vi "HMI Respirador.vi"() -> ()   [LabVIEW 2019]
uses:
  <vilib>/Instr/_visa.llb/VISA Configure Serial Port (Instr).vi
panel:
  in  "byte count":u32
  out "Waveform Chart":dynamicdata(graph)
  out "V. Espir.":bool
  out "V.Aspir":bool
  out "Boolean 3":bool
  out "Trama de Datos":string
  out "Meter":dbl(knob) scale=0.0..10.0
  out "VENTILADOR":bool
  out "TUBERIA EXHALACION":u8(slide)
  out "TUBERIA INHALACION":u8(slide) scale=0.0..115.0
  in  "stop":bool
  out "Velocidad Motor  R.P.M":i32
  out "Presion Entregada":i32
  in  "write buffer":string
  in  "Tiempo PEEP":u16
  out "read buffer":string
  out "Boolean":bool
  in  "Guardar Config":bool
  in  "Iniciar":bool
  in  "Puerto Comunicación":refnum<visa-resource-name>
  in  "Presión Maxima":u8
  in  "PEEP (pres. esp.)":u8
  in  "Tiempo Anspiracion":u16
  in  "Turbina %":u8
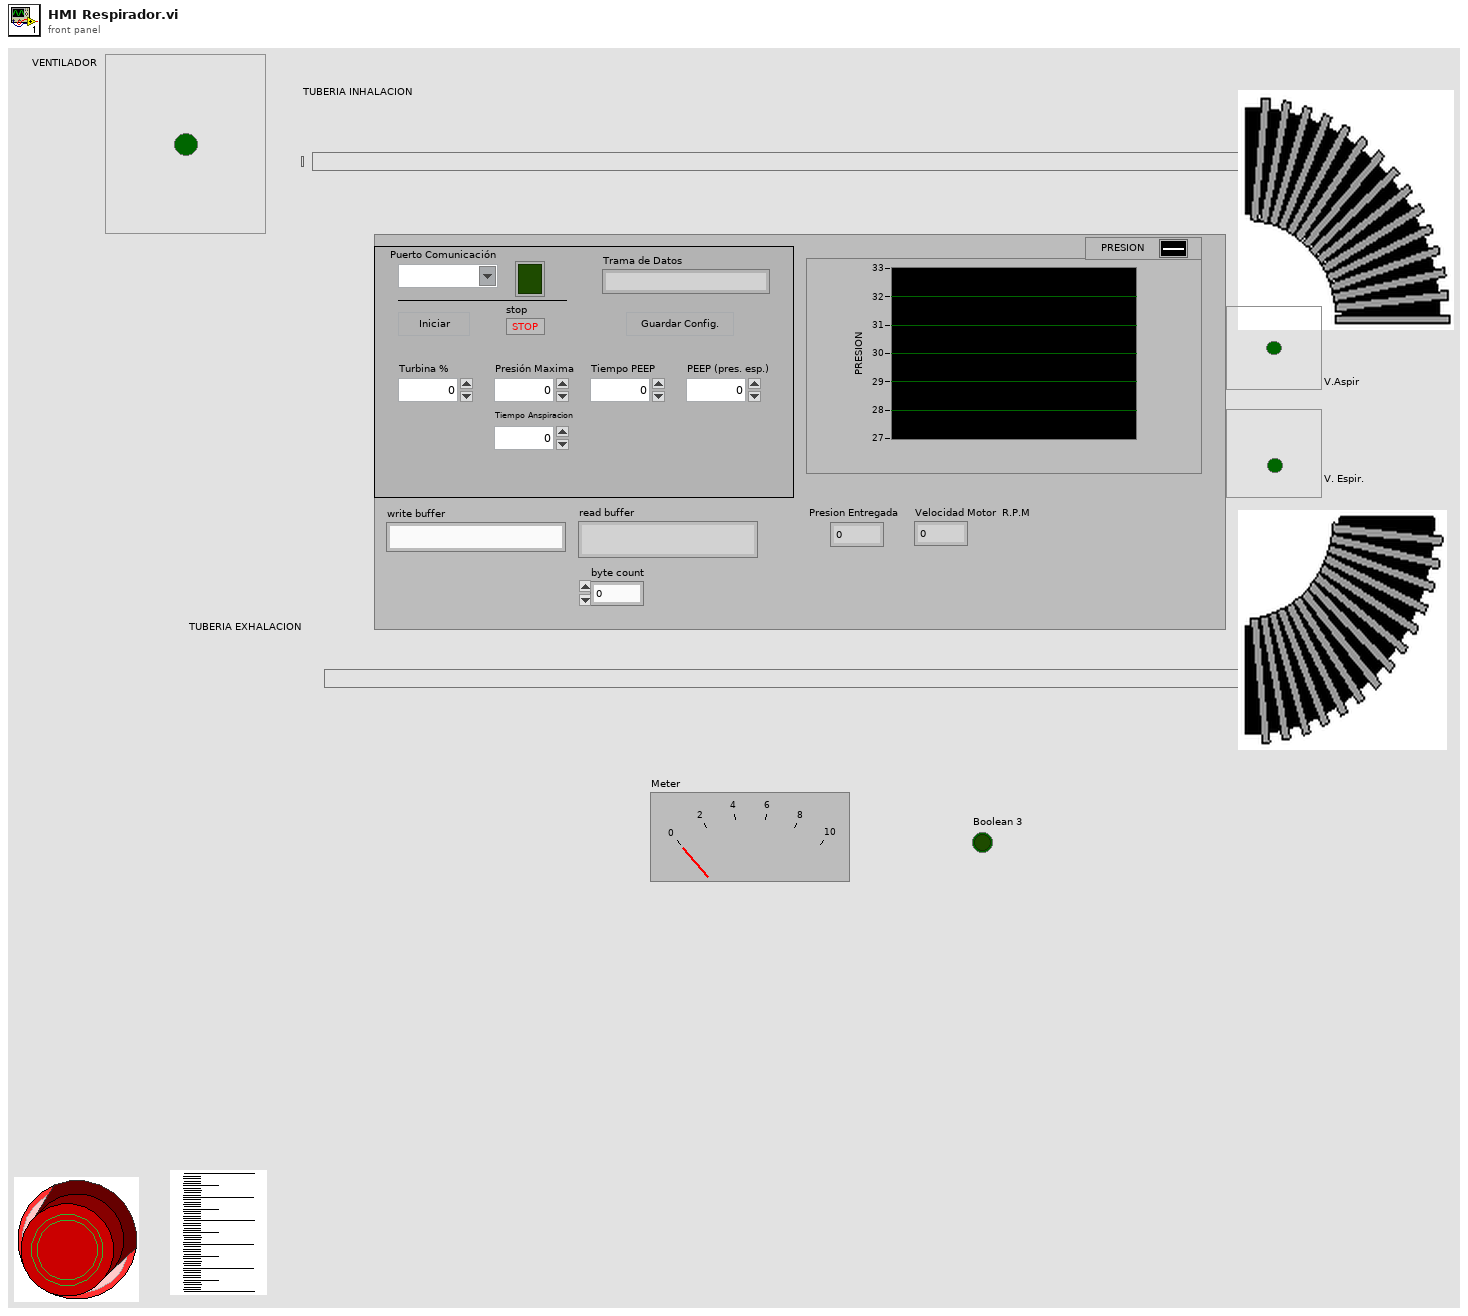
[diagram p1: front panel]
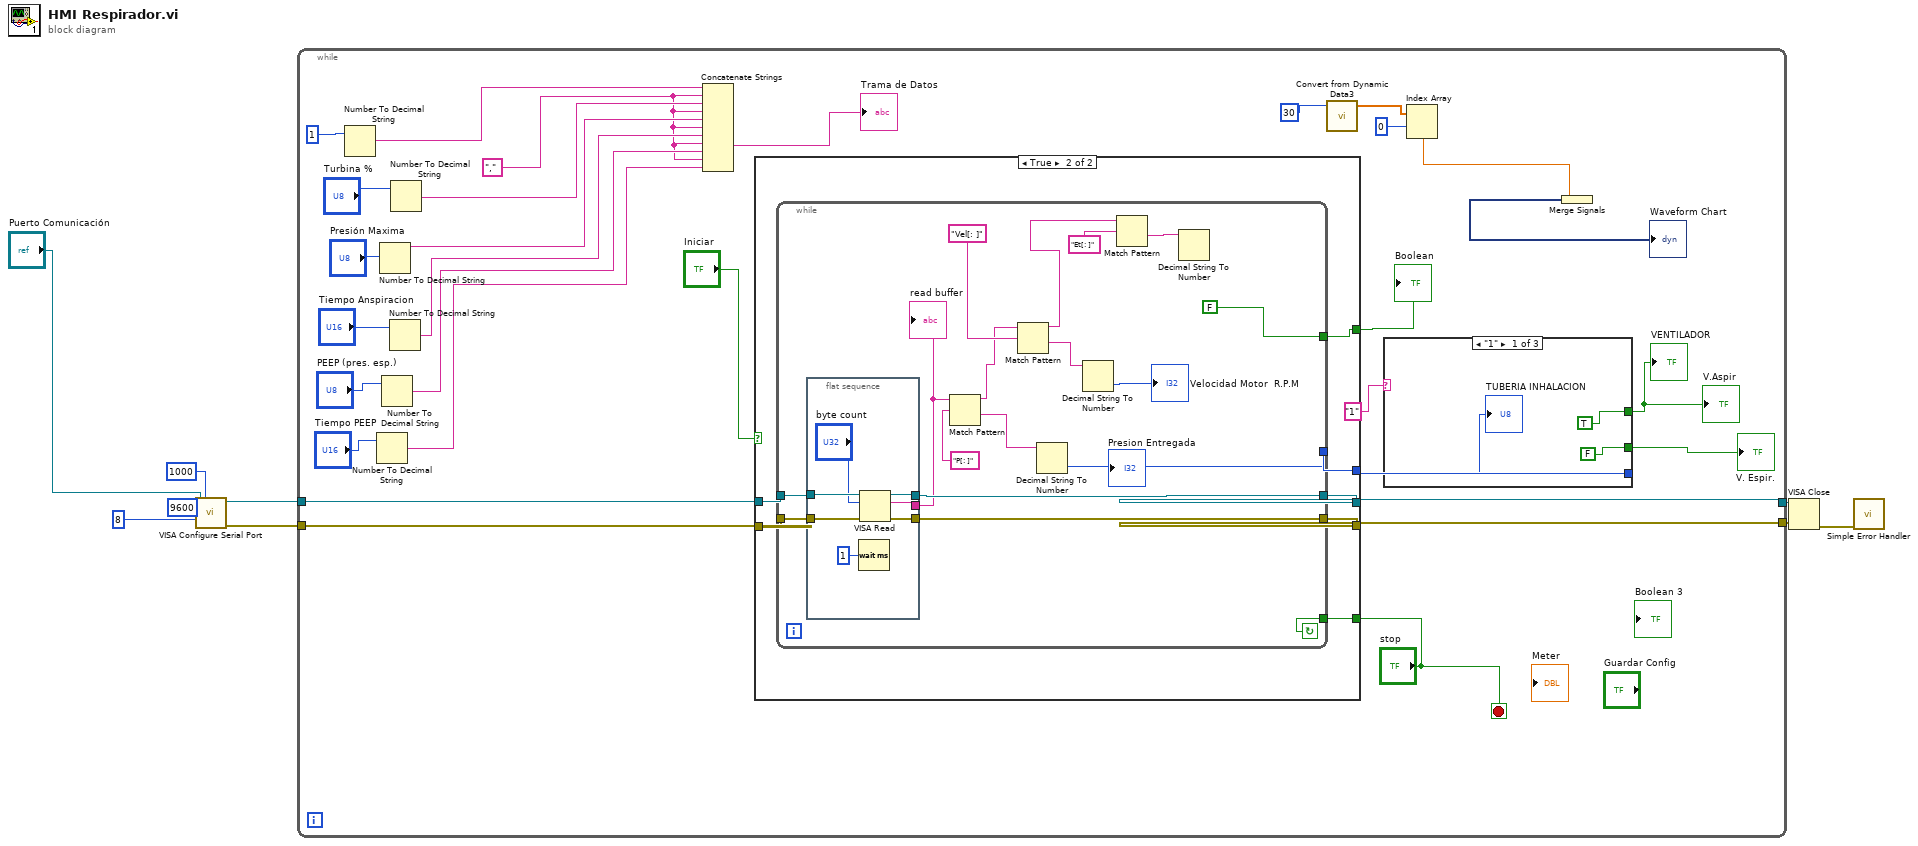
[diagram p0: block diagram]
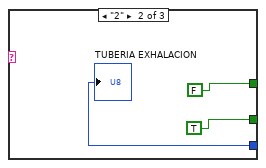
[diagram p2: hidden frame]
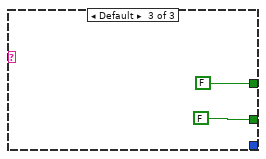
[diagram p3: hidden frame]
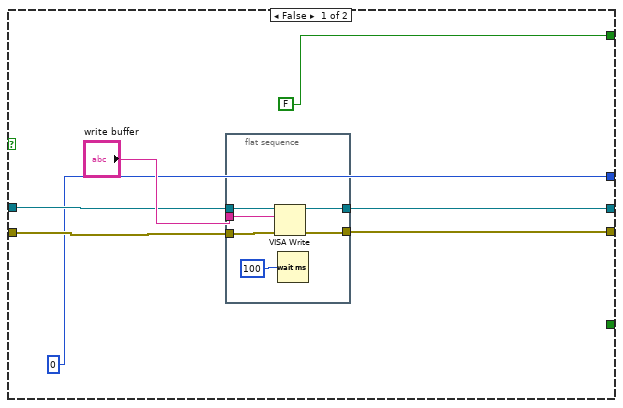
[diagram p4: hidden frame]
diagram:
  n1 = call-poly "VISA Configure Serial Port"("VISA resource name"="Puerto Comunicación", "timeout (10sec)"=u32 1000, "baud rate (9600)"=u32 9600, "data bits (8)"=u16 8) -> ("VISA resource name out"=w8:refnum<visa-resource-name>, "error out"=w7:errorcluster)  [unwired: 5 in, 5 out]
  n2 = while {
    tunnel: w8 -> [w37]
    tunnel: w7 -> [w38]
    tunnel: [w36] -> w4
    tunnel: [w35] -> w3
    stop <- "stop" stop-if-true
    w26 = ","
    n3 = Number To Decimal String(number=1) -> (decimal integer string=w31:string)  [unwired: 1 in]
    n4 = Number To Decimal String(number="Tiempo PEEP") -> (decimal integer string=w25:string)  [unwired: 1 in]
    n5 = Number To Decimal String(number="Presión Maxima") -> (decimal integer string=w29:string)  [unwired: 1 in]
    n6 = Number To Decimal String(number="PEEP (pres. esp.)") -> (decimal integer string=w27:string)  [unwired: 1 in]
    n7 = Number To Decimal String(number="Tiempo Anspiracion") -> (decimal integer string=w28:string)  [unwired: 1 in]
    n8 = Number To Decimal String(number="Turbina %") -> (decimal integer string=w30:string)  [unwired: 1 in]
    n9 = Concatenate Strings(w31, w26, w30, w26, w29, w26, w28, w26, w27, w26, w25) -> (→"Trama de Datos":string)
    n10 = case shown="True" "Iniciar" {
      tunnel: w37 -> [w51 w67]
      tunnel: w38 -> [w50 w66]
      tunnel: [w53 w65] -> w36
      tunnel: [w52 w64] -> w35
      tunnel: [FALSE w63] -> w23
      tunnel: "stop" -> [_ w62]
      tunnel: [0 w61] -> w18
      frame False {
        n11 = flat-sequence {
          tunnel: w51 -> [w60]
          tunnel: w50 -> [w59]
          tunnel: "write buffer" -> [w58]
          tunnel: [w57] -> w53
          tunnel: [w56] -> w52
          frame #0 {
            n12 = VISA Write(VISA resource name=w60, write buffer=w58, error in (no error)=w59) -> (VISA resource name out=w57:refnum<visa-resource-name>, error out=w56:errorcluster)  [unwired: 1 out]
            n13 = Wait (ms)(milliseconds to wait=u32 100) -> ()  [unwired: 1 out]
          }
        }
      }
      frame True {
        n14 = while {
          tunnel: w67 -> [w84]
          tunnel: [w82] -> w65
          tunnel: w66 -> [w83]
          tunnel: [w81] -> w64
          tunnel: [FALSE] -> w63
          tunnel: w62 -> [w72]
          tunnel: [w68] -> w61
          stop <- w72 continue-if-true
          n15 = flat-sequence {
            tunnel: w84 -> [w91]
            tunnel: w83 -> [w90]
            tunnel: [w89] -> w82
            tunnel: [w88] -> w81
            tunnel: [w87] -> w76
            frame #0 {
              n16 = Wait (ms)(milliseconds to wait=u32 1) -> ()  [unwired: 1 out]
              n17 = VISA Read(VISA resource name=w91, byte count="byte count", error in (no error)=w90) -> (VISA resource name out=w89:refnum<visa-resource-name>, read buffer=w87:string, error out=w88:errorcluster)  [unwired: 1 out]
            }
          }
          n18 = Match Pattern(string=w76, regular expression="P[: ]") -> (before substring=w74:string, after substring=w79:string)  [unwired: 1 in, 2 out]
          n19 = Match Pattern(string=w74, regular expression="Vel[: ]") -> (before substring=w71:string, after substring=w75:string)  [unwired: 1 in, 2 out]
          n20 = Decimal String To Number(string=w79) -> (number=w68:i32)  [unwired: 2 in, 1 out]
          "Presion Entregada" <- w68
          n21 = Decimal String To Number(string=w75) -> (number=→"Velocidad Motor  R.P.M":i32)  [unwired: 2 in, 1 out]
          n22 = Match Pattern(string=w71, regular expression="Et[: ]") -> (after substring=w69:string)  [unwired: 1 in, 3 out]
          n23 = Decimal String To Number(string=w69) -> ()  [unwired: 2 in, 2 out]
          "read buffer" <- w76
        }
      }
    }
    "Boolean" <- w23
    n24 = call "Convert from Dynamic Data3"("Dynamic Data Type"=30) -> ("Array"=w10:dbl[])  [unwired: 3 in]
    n25 = case shown="\"1\"" "1" {
      tunnel: w18 -> [w41 w44 _]
      tunnel: [TRUE FALSE FALSE] -> w16
      tunnel: [FALSE TRUE FALSE] -> w15
      frame "1" {
        "TUBERIA INHALACION" <- w41
      }
      frame "2" {
        "TUBERIA EXHALACION" <- w44
      }
      frame Default {
      }
    }
    "VENTILADOR" <- w16
    "V.Aspir" <- w16
    "V. Espir." <- w15
    n26 = Index Array(array=w10, index #1=0 ("index")) -> (element #1=w12:dbl)  [unwired: 1 in, 1 out]
    n27 = Merge Signals(w12) -> (→"Waveform Chart":dynamicdata)
  }
  n28 = VISA Close(VISA resource name=w4, error in (no error)=w3) -> (error out=w9:errorcluster)
  n29 = call <vilib>:"Simple Error Handler.vi"("error in (no error)"=w9) -> ()  [unwired: 1 in, 8 out]
